vi "Make camera cluster.vi"(8 "Error In":errorcluster, 9 "Blue ref":refnum<k24>, 10 "Green ref":refnum<k24>, 11 "Red ref":refnum<k24>) -> (0 "Error Out":errorcluster, 3 "Camera cluster":T1)   [LabVIEW 2017]
uses:
  C:/Program Files/National Instruments/LabVIEW 2017/instr.lib/IDS/ueye.NET/uEyeDotNet.dll
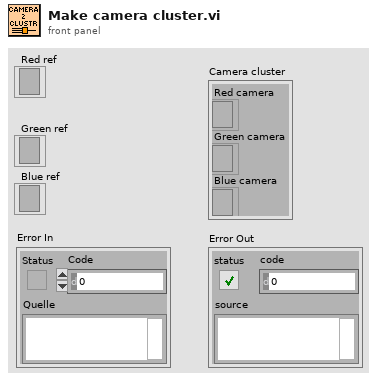
[diagram p1: front panel]
types:
  T1 = cluster{"Red camera":refnum<k24>, "Green camera":refnum<k24>, "Blue camera":refnum<k24>}
  T2 = cluster{"Blue camera":refnum<k24>, "Green camera":refnum<k24>, "Red camera":refnum<k24>}
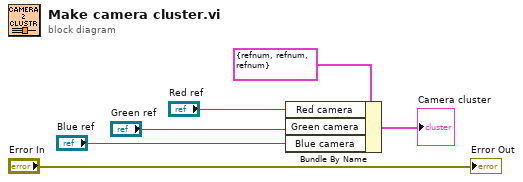
[diagram p0: block diagram]
diagram:
  n1 = Bundle By Name(cluster=T2 {"Blue camera"=refnum, "Green camera"=refnum, "Red camera"=refnum} ("input cluster"), "Red camera"="Red ref", "Green camera"="Green ref", "Blue camera"="Blue ref") -> (→"Camera cluster":T2)
  "Error Out" <- "Error In"
